vi "Example TIF Read.vi"() -> ()   [LabVIEW 2016]
uses:
  ImageJ TIF Type Defs/TIF Read Image Information.ctl
panel:
  out "Image Info":T1
  out "Image Stack":u16[][][](array[numeric])
  in  "TIF Image":path
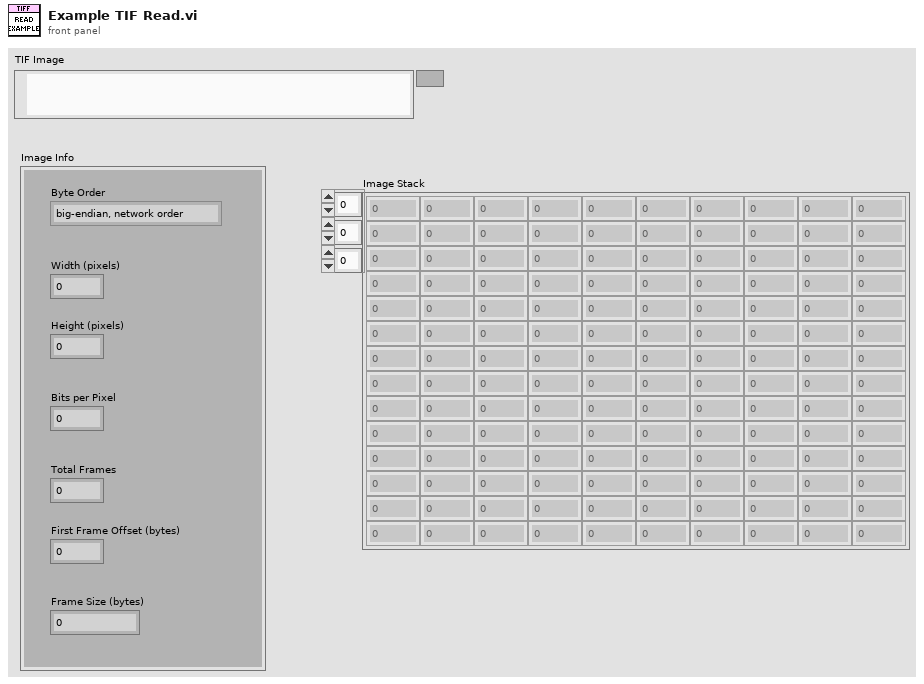
[diagram p1: front panel]
types:
  T1 = typedef "TIF Read Image Information.ctl" = cluster{"Byte Order":enum16{"big-endian, network order", "native, host order", "little-endian"}, "Width (pixels)":i32, "Height (pixels)":i32, "Bits per Pixel":u8, "Total Frames":u32, "First Frame Offset (bytes)":u32, "Frame Size (bytes)":u32}
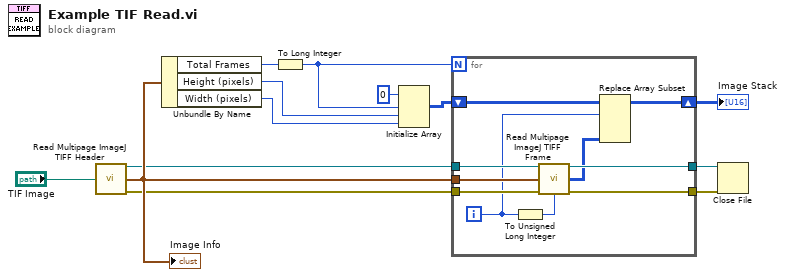
[diagram p0: block diagram]
diagram:
  n1 = call "Read Multipage ImageJ TIFF Header.vi"("TIFF Path"="TIF Image") -> ("TIF Ref"=w8:refnum<file>, "Image Info"=w10:T1, "Error"=w9:errorcluster)  [unwired: 12 in]
  "Image Info" <- w10
  n2 = Unbundle By Name(w10) -> ("Total Frames"=w11:u32, "Height (pixels)"=w4:i32, "Width (pixels)"=w3:i32)
  n3 = To Long Integer(number=w11) -> (32bit integer=w2:i32)
  n4 = Initialize Array(u16 0 ("element"), w2, w4, w3) -> (w12:u16[][][])
  n5 = for {
    N: w2 -> [_]
    tunnel: w8 -> [w23]
    tunnel: w10 -> [w22]
    tunnel: w9 -> [w21]
    shift-right: [w16] -> w1
    shift-left: w12 -> [w17]
    tunnel: [w19] -> w13
    tunnel: [w18] -> w6
    i -> [w15]
    n6 = To Unsigned Long Integer(number=w15) -> (unsigned 32bit integer=w20:u32)
    n7 = call "Read Multipage ImageJ TIFF Frame.vi"("TIF Ref"=w23, "Image Info"=w22, "Error"=w21, "Frame"=w20) -> ("TIF Ref (Dup)"=w19:refnum<file>, "U16 Image"=w14:u16[][], "Error"=w18:errorcluster)  [unwired: 8 in, 1 out]
    n8 = Replace Array Subset(array=w17, new element=w14, index (dim 0)=w15) -> (w16:u16[][][])  [unwired: 2 in]
  }
  "Image Stack" <- w1
  n9 = Close File(refnum=w13, error in=w6) -> ()  [unwired: 2 out]
